vi "Array practice problem 3.vi"() -> ()   [LabVIEW 2018]
panel:
  out "Array":i32[](array[numeric])
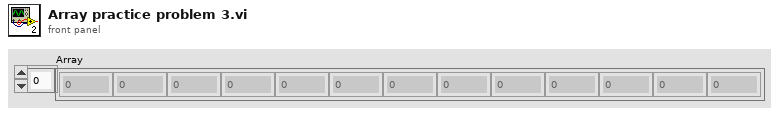
[diagram p1: front panel]
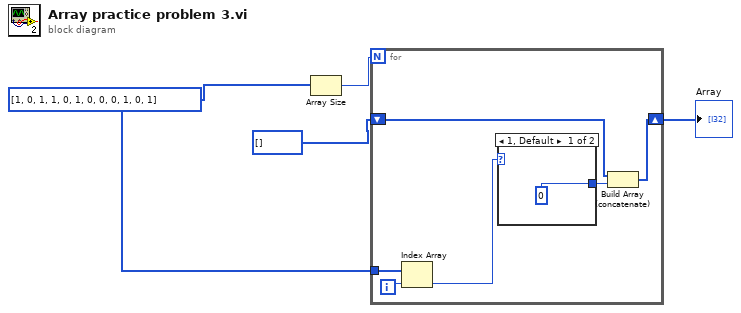
[diagram p0: block diagram]
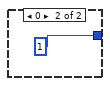
[diagram p2: hidden frame]
diagram:
  w3 = i32[] [1, 0, 1, 1, 0, 1, 0, 0, 0, 1, 0, 1]
  n1 = Array Size(array=w3) -> (size(s)=w4:i32)
  n2 = for {
    N: w4 -> [_]
    tunnel: w3 -> [w9]
    shift-right: [w5] -> w1
    shift-left: i32[] [] -> [w7]
    i -> [w10]
    n3 = Index Array(array=w9, index=w10) -> (element=w8:i32)
    n4 = case shown="1, Default" w8 {
      tunnel: [0 1] -> w6
      frame 1, Default {
      }
      frame 0 {
      }
    }
    n5 = Build Array (concatenate)(w7, w6) -> (w5:i32[])
  }
  "Array" <- w1
